vi "DAC.vi"() -> ()   [LabVIEW 2024]
uses:
  <vilib>/measure/NI_MABase.lvlib
panel:
  in  "Offset [V]":dbl
  out "quantization error":dbl
  out "decimal value":dbl
  in  "max [V]":dbl
  in  "min [V]":dbl
  in  "Number of bits":dbl
  out "Sampled Signal":waveform(dbl)(graph)
  out "Original Signal":waveform(dbl)(graph)
  in  "Sampling Frequency [Hz]":dbl
  in  "Type of signal":T1(ring)
  in  "Amplitude [V]":dbl
  in  "Frequency [Hz]":dbl
  out "bit value":bool[](array[boolean])
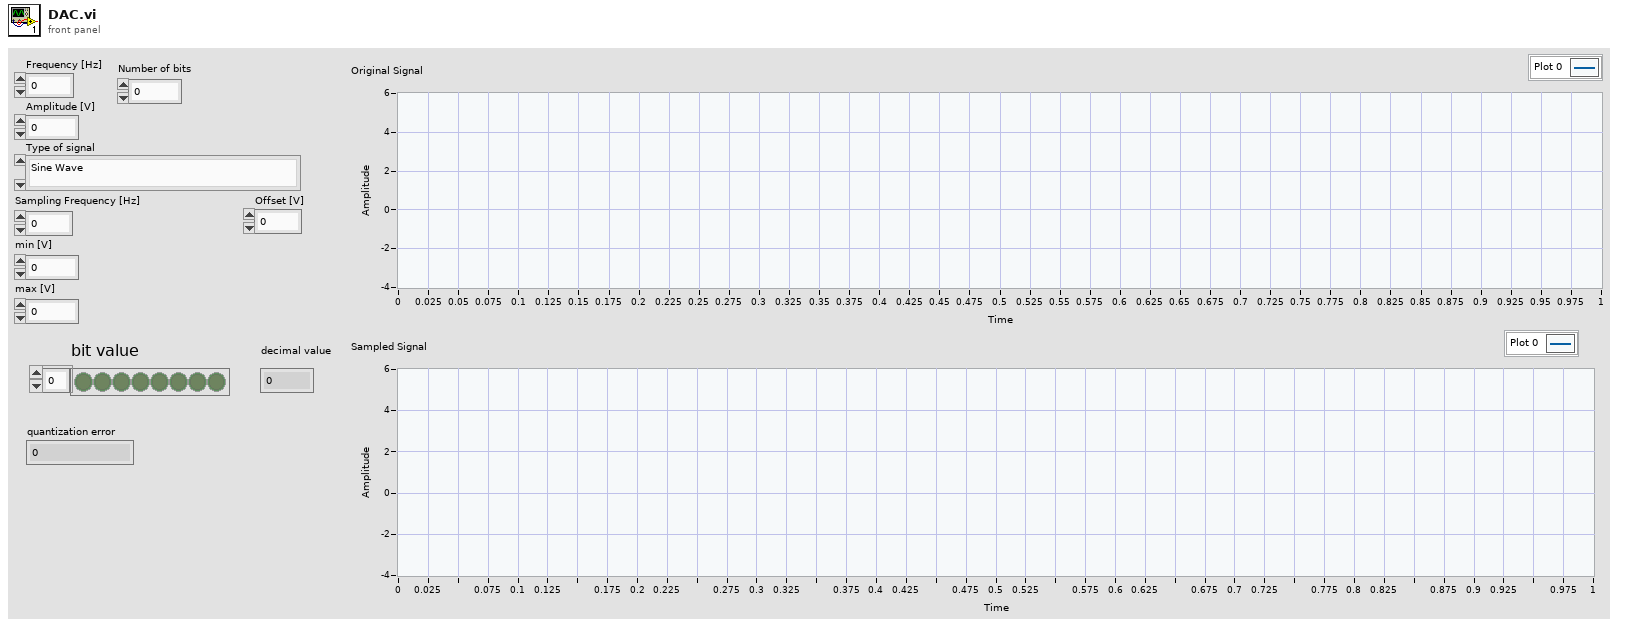
[diagram p1: front panel]
types:
  T1 = enum16{"Sine Wave", "Triangle Wave", "Square Wave", "Sawtooth Wave"}
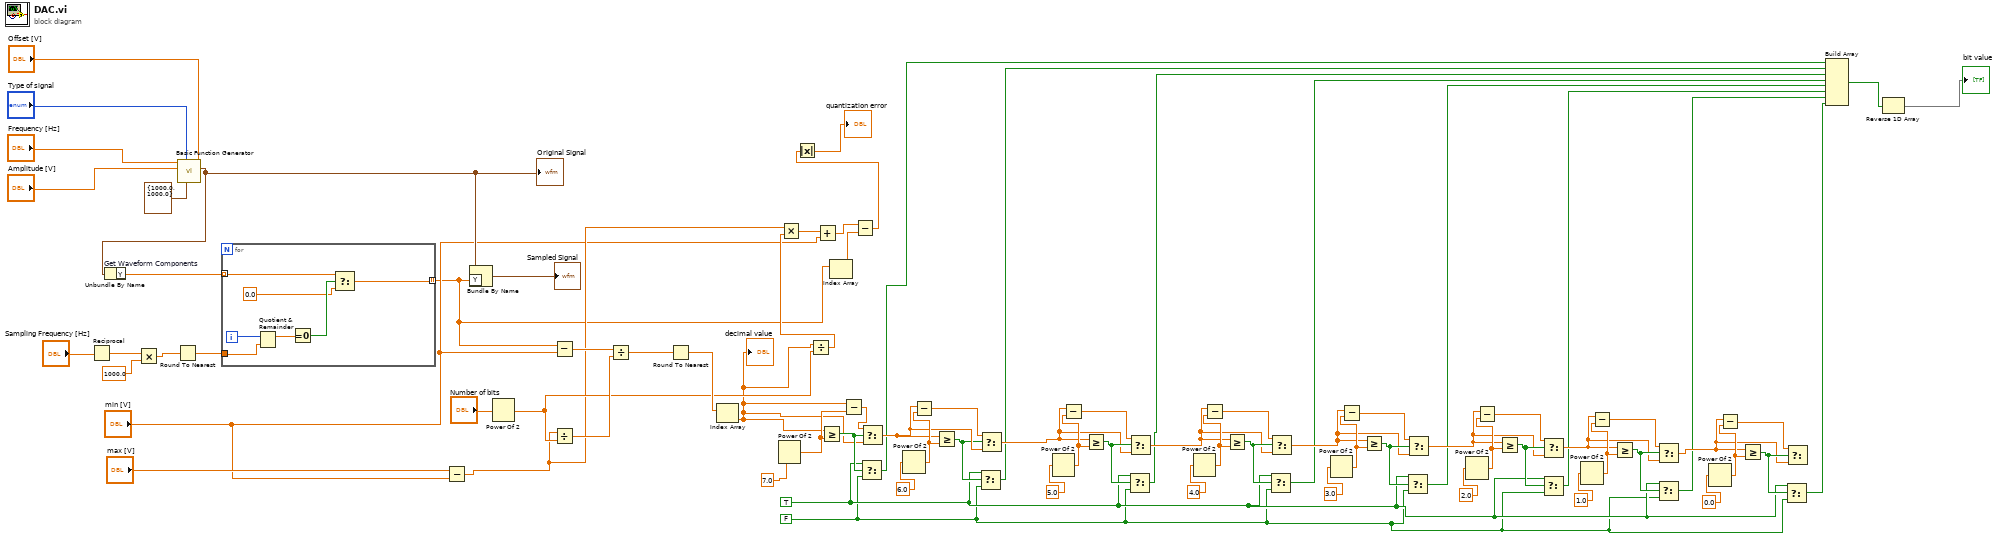
[diagram p0: block diagram]
diagram:
  w23 = FALSE
  w24 = TRUE
  n1 = Reciprocal(x="Sampling Frequency [Hz]") -> (1/x=w71:dbl)
  n2 = Multiply(x=w71, y=1000.0) -> (x*y=w13:dbl)
  n3 = Round To Nearest(number=w13) -> (nearest integer value=w12:dbl)
  n4 = call <vilib>:"Basic Function Generator.vi"("offset"="Offset [V]", "sampling info"=cluster{"Fs":dbl, "#s":dbl} {"Fs"=1000.0, "#s"=1000.0}, "signal type"="Type of signal", "amplitude"="Amplitude [V]", "frequency"="Frequency [Hz]") -> ("signal out"=w70:waveform(dbl))  [unwired: 4 in, 2 out]
  "Original Signal" <- w70
  n5 = Unbundle By Name "Get Waveform Components"(w70) -> ("Y"=w76:dbl[])
  n6 = for {
    tunnel: w76 -> [w84] mode=indexing
    tunnel: w12 -> [w87]
    tunnel: [w82] -> w16 mode=indexing
    i -> [w88]
    n7 = Quotient & Remainder(x=w88, y=w87) -> (x-y*floor(x/y)=w86:dbl)  [unwired: 1 out]
    n8 = Equal To 0?(x=w86) -> (x = 0?=w85:bool)
    n9 = Select(t=w84, s=w85, f=0.0) -> (s? t:f=w82:dbl)
  }
  n10 = Subtract(x="max [V]", y="min [V]") -> (x-y=w19:dbl)
  n11 = Bundle By Name(cluster=w70, "Y"=w16) -> (→"Sampled Signal":waveform(dbl))
  n12 = Power Of 2(x="Number of bits") -> (2^x=w22:dbl)
  n13 = Subtract(x=w16, y="min [V]") -> (x-y=w69:dbl[])
  n14 = Divide(x=w19, y=w22) -> (x/y=w66:dbl)
  n15 = Divide(x=w69, y=w66) -> (x/y=w65:dbl[])
  n16 = Round To Nearest(number=w65) -> (nearest integer value=w64:dbl[])
  n17 = Index Array(array=w64) -> (element=w21:dbl)  [unwired: 1 in]
  "decimal value" <- w21
  n18 = Power Of 2(x=7.0 ("y")) -> (2^x=w62:dbl)
  n19 = Divide(x=w21, y=w22) -> (x/y=w20:dbl)
  n20 = Multiply(x=w19, y=w20) -> (x*y=w18:dbl)
  n21 = Add(x=w18, y="min [V]") -> (x+y=w14:dbl)
  n22 = Greater Or Equal?(x=w21, y=w62) -> (x >= y?=w60:bool)
  n23 = Index Array(array=w16) -> (element=w15:dbl)  [unwired: 1 in]
  n24 = Subtract(x=w21, y=w62) -> (x-y=w61:dbl)
  n25 = Subtract(x=w14, y=w15) -> (x-y=w3:dbl)
  n26 = Absolute Value(x=w3) -> (abs(x)=→"quantization error":dbl)
  n27 = Select(t=w24, s=w60, f=w23) -> (s? t:f=w11:bool)
  n28 = Select(t=w61, s=w60, f=w21) -> (s? t:f=w56:dbl)
  n29 = Power Of 2(x=6.0 ("y")) -> (2^x=w58:dbl)
  n30 = Subtract(x=w56, y=w58) -> (x-y=w57:dbl)
  n31 = Greater Or Equal?(x=w56, y=w58) -> (x >= y?=w55:bool)
  n32 = Select(t=w24, s=w55, f=w23) -> (s? t:f=w10:bool)
  n33 = Select(t=w57, s=w55, f=w56) -> (s? t:f=w50:dbl)
  n34 = Power Of 2(x=5.0 ("y")) -> (2^x=w53:dbl)
  n35 = Subtract(x=w50, y=w53) -> (x-y=w52:dbl)
  n36 = Greater Or Equal?(x=w50, y=w53) -> (x >= y?=w51:bool)
  n37 = Select(t=w24, s=w51, f=w23) -> (s? t:f=w9:bool)
  n38 = Select(t=w52, s=w51, f=w50) -> (s? t:f=w45:dbl)
  n39 = Power Of 2(x=4.0 ("y")) -> (2^x=w48:dbl)
  n40 = Subtract(x=w45, y=w48) -> (x-y=w47:dbl)
  n41 = Greater Or Equal?(x=w45, y=w48) -> (x >= y?=w46:bool)
  n42 = Select(t=w24, s=w46, f=w23) -> (s? t:f=w8:bool)
  n43 = Select(t=w47, s=w46, f=w45) -> (s? t:f=w40:dbl)
  n44 = Power Of 2(x=3.0 ("y")) -> (2^x=w43:dbl)
  n45 = Subtract(x=w40, y=w43) -> (x-y=w42:dbl)
  n46 = Greater Or Equal?(x=w40, y=w43) -> (x >= y?=w41:bool)
  n47 = Select(t=w24, s=w41, f=w23) -> (s? t:f=w7:bool)
  n48 = Select(t=w42, s=w41, f=w40) -> (s? t:f=w35:dbl)
  n49 = Power Of 2(x=2.0 ("y")) -> (2^x=w38:dbl)
  n50 = Subtract(x=w35, y=w38) -> (x-y=w37:dbl)
  n51 = Greater Or Equal?(x=w35, y=w38) -> (x >= y?=w36:bool)
  n52 = Select(t=w24, s=w36, f=w23) -> (s? t:f=w6:bool)
  n53 = Select(t=w37, s=w36, f=w35) -> (s? t:f=w30:dbl)
  n54 = Power Of 2(x=1.0 ("y")) -> (2^x=w33:dbl)
  n55 = Subtract(x=w30, y=w33) -> (x-y=w32:dbl)
  n56 = Greater Or Equal?(x=w30, y=w33) -> (x >= y?=w31:bool)
  n57 = Select(t=w24, s=w31, f=w23) -> (s? t:f=w5:bool)
  n58 = Select(t=w32, s=w31, f=w30) -> (s? t:f=w25:dbl)
  n59 = Power Of 2(x=0.0 ("y")) -> (2^x=w28:dbl)
  n60 = Subtract(x=w25, y=w28) -> (x-y=w27:dbl)
  n61 = Greater Or Equal?(x=w25, y=w28) -> (x >= y?=w26:bool)
  n62 = Select(t=w24, s=w26, f=w23) -> (s? t:f=w4:bool)
  n63 = Select(t=w27, s=w26, f=w25) -> ()  [unwired: 1 out]
  n64 = Build Array(w11, w10, w9, w8, w7, w6, w5, w4) -> (w81:bool[])
  n65 = Reverse 1D Array(array=w81) -> (reversed array=→"bit value":bool[])
